vi "Преобразователь 2-10 в доп.vi"(1 "-":bool, 2 "H":T2, 3 "L":T3) -> (0 "R":T1)   [LabVIEW 2017]
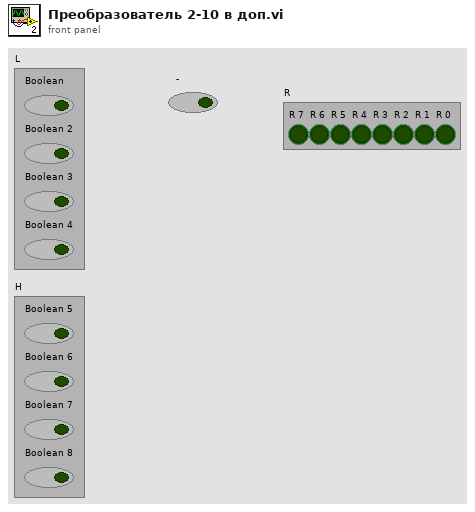
[diagram p1: front panel]
types:
  T1 = cluster{"R 7":bool, "R 6":bool, "R 5":bool, "R 4":bool, "R 3":bool, "R 2":bool, "R 1":bool, "R 0":bool}
  T2 = cluster{"Boolean 5":bool, "Boolean 6":bool, "Boolean 7":bool, "Boolean 8":bool}
  T3 = cluster{"Boolean":bool, "Boolean 2":bool, "Boolean 3":bool, "Boolean 4":bool}
  T4 = cluster{"Si":bool, "Si":bool, "Si":bool, "Si":bool, "Si":bool, "Si":bool, "Si":bool, "Si":bool}
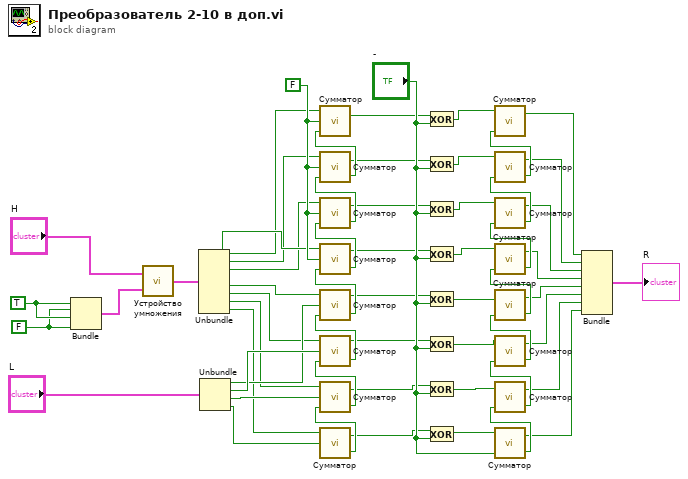
[diagram p0: block diagram]
diagram:
  w43 = FALSE
  w57 = FALSE
  w58 = TRUE
  n1 = Bundle(w58, w57, w58, w57) -> (w56:cluster{bool, bool, bool, bool})  [unwired: 1 in]
  n2 = call "Устройство умножения.vi"("B"=w56, "A"="H") -> ("R"=w55:T1)
  n3 = Unbundle(w55) -> ("R 7"=w35:bool, "R 6"=w36:bool, "R 5"=w37:bool, "R 4"=w38:bool, "R 3"=w39:bool, "R 2"=w40:bool, "R 1"=w41:bool, "R 0"=w42:bool)
  n4 = Unbundle("L") -> ("Boolean"=w51:bool, "Boolean 2"=w52:bool, "Boolean 3"=w53:bool, "Boolean 4"=w54:bool)
  n5 = call "Сумматор.vi"("B"=w54, "A"=w42) -> ("Ci"=w50:bool, "Si"=w17:bool)  [unwired: 1 in]
  n6 = call "Сумматор.vi"("i-1"=w50, "B"=w53, "A"=w41) -> ("Ci"=w49:bool, "Si"=w16:bool)
  n7 = call "Сумматор.vi"("i-1"=w49, "B"=w52, "A"=w40) -> ("Ci"=w48:bool, "Si"=w15:bool)
  n8 = call "Сумматор.vi"("i-1"=w48, "B"=w51, "A"=w39) -> ("Ci"=w47:bool, "Si"=w14:bool)
  n9 = call "Сумматор.vi"("i-1"=w47, "B"=w43, "A"=w38) -> ("Ci"=w46:bool, "Si"=w13:bool)
  n10 = call "Сумматор.vi"("i-1"=w46, "B"=w43, "A"=w37) -> ("Ci"=w45:bool, "Si"=w12:bool)
  n11 = call "Сумматор.vi"("i-1"=w45, "B"=w43, "A"=w36) -> ("Ci"=w44:bool, "Si"=w11:bool)
  n12 = call "Сумматор.vi"("i-1"=w44, "B"=w43, "A"=w35) -> ("Si"=w10:bool)  [unwired: 1 out]
  n13 = Exclusive Or(1:"-", 2:w10) -> (0:w33:bool)
  n14 = Exclusive Or(1:"-", 2:w11) -> (0:w32:bool)
  n15 = Exclusive Or(1:"-", 2:w12) -> (0:w31:bool)
  n16 = Exclusive Or(1:"-", 2:w13) -> (0:w30:bool)
  n17 = Exclusive Or(1:"-", 2:w14) -> (0:w29:bool)
  n18 = Exclusive Or(1:"-", 2:w15) -> (0:w28:bool)
  n19 = Exclusive Or(1:"-", 2:w16) -> (0:w27:bool)
  n20 = Exclusive Or(1:"-", 2:w17) -> (0:w26:bool)
  n21 = call "Сумматор.vi"("i-1"="-", "A"=w26) -> ("Ci"=w24:bool, "Si"=w1:bool)  [unwired: 1 in]
  n22 = call "Сумматор.vi"("i-1"=w24, "A"=w27) -> ("Ci"=w23:bool, "Si"=w2:bool)  [unwired: 1 in]
  n23 = call "Сумматор.vi"("i-1"=w23, "A"=w28) -> ("Ci"=w22:bool, "Si"=w3:bool)  [unwired: 1 in]
  n24 = call "Сумматор.vi"("i-1"=w22, "A"=w29) -> ("Ci"=w21:bool, "Si"=w4:bool)  [unwired: 1 in]
  n25 = call "Сумматор.vi"("i-1"=w21, "A"=w30) -> ("Ci"=w20:bool, "Si"=w5:bool)  [unwired: 1 in]
  n26 = call "Сумматор.vi"("i-1"=w20, "A"=w31) -> ("Ci"=w19:bool, "Si"=w6:bool)  [unwired: 1 in]
  n27 = call "Сумматор.vi"("i-1"=w19, "A"=w32) -> ("Ci"=w18:bool, "Si"=w7:bool)  [unwired: 1 in]
  n28 = call "Сумматор.vi"("i-1"=w18, "A"=w33) -> ("Si"=w8:bool)  [unwired: 1 in, 1 out]
  n29 = Bundle("Si"=w8, "Si"=w7, "Si"=w6, "Si"=w5, "Si"=w4, "Si"=w3, "Si"=w2, "Si"=w1) -> (→"R":T4)  [unwired: 1 in]
